vi "GEOM_Geom2Str.vi"(8 "error in (no error)":errorcluster) -> (0 "error out":errorcluster, 1 "geometry command":string, 2 "binning command":string)   [LabVIEW 2016]
uses:
  GEOM_VAR_action.ctl
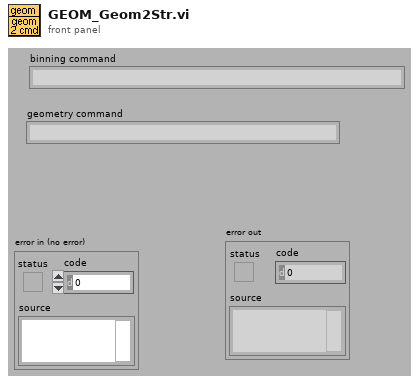
[diagram p1: front panel]
types:
  T1 = typedef "GEOM_VAR_action.ctl" = enum16{"read", "write"}
  T2 = typedef "GEOM_AmpModifiers.ctl" = cluster{"Binning":T3, "sections":T4[]}
  T3 = typedef "GEOM_Binning.ctl" = cluster{"x":u32, "y":u32}
  T4 = typedef "GEOM_Moifier.ctl" = cluster{"name":string, "header section":string, "comment":string, "value":i32, "binning?":bool, "Where":enum16{"predata", "postdata"}, "add In":enum16{"columns", "rows", "none"}}
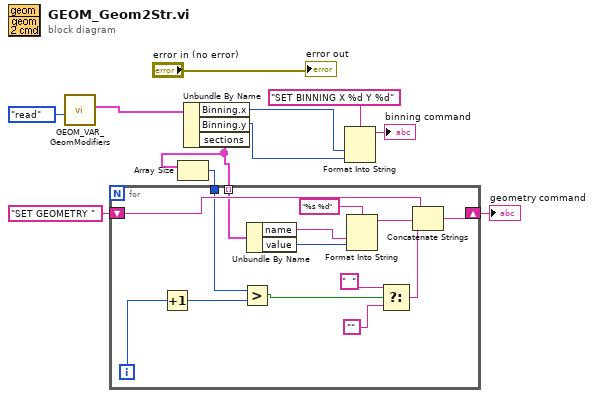
[diagram p0: block diagram]
diagram:
  n1 = call "GEOM_VAR_GeomModifiers.vi"("Action"=GEOM_VAR_action."read") -> ("GEOM_modifiers out"=w2:T2)  [unwired: 1 in, 9 out]
  n2 = Unbundle By Name(w2) -> ("Binning.x"=w10:u32, "Binning.y"=w9:u32, "sections"=w6:T4[])
  n3 = Array Size(array=w6) -> (size(s)=w5:i32)
  n4 = for {
    tunnel: w6 -> [w19] mode=indexing
    shift-right: [w21] -> w4
    shift-left: "SET GEOMETRY " -> [w20]
    tunnel: w5 -> [w18]
    i -> [w17]
    n5 = Increment(x=w17) -> (x+1=w12:i32)
    n6 = Greater?(x=w18, y=w12) -> (0:w16:bool)
    n7 = Unbundle By Name(w19) -> ("name"=w24:string, "value"=w23:i32)
    n8 = Format Into String(format string="%s %d", w24, w23) -> (resulting string=w22:string)  [unwired: 2 in, 1 out]
    n9 = Select(t="  ", s=w16, f="") -> (s? t:f=w14:string)
    n10 = Concatenate Strings(w20, w22, w14) -> (w21:string)
  }
  "geometry command" <- w4
  n11 = Format Into String(format string="SET BINNING X %d Y %d", w10, w9) -> (resulting string=→"binning command":string)  [unwired: 2 in, 1 out]
  "error out" <- "error in (no error)"
